vi "Verify.vi"(8 "error in (no error)":errorcluster, 9 "Issuer URI path (component)":string, 10 "Client ID":string, 11 "JSONWebToken in":refnum<class "JSONWebToken.lvclass">) -> (0 "error out":errorcluster, 2 "Valid JWT?":bool, 3 "JSONWebToken out":refnum<class "JSONWebToken.lvclass">)   [LabVIEW 2020, in "JSONWebToken.lvclass"]
doc: "https://openid.net/specs/openid-connect-basic-1_0.html#IDTokenValidation\n\nThe Client MUST validate the ID Token in the Token Response. To do this, the Client can split the ID Token at the period (\".\") characters, take the second segment, and base64url decode it to obtain a JSON object containing the ID Token Claims, which MUST be validated as follows:\n\nThe Issuer Identifier for the OpenID Provider (which is typically obtained during Discovery) MUST exactly match the value of the iss (issuer) Claim.\n\nThe Client MUST validate that the aud (audience) Claim contains its client_id value registered at the Issuer identified by the iss (issuer) Claim as an audience. The ID Token MUST be rejected if the ID Token does not list the Client as a valid audience, or if it contains additional audiences not trusted by the Client.\n\nThe current time MUST be before the time represented by the exp Claim (possibly allowing for some small leeway to account for clock skew).\n\nThe iat Claim can be used to reject tokens that were issued too far away from the current time, limiting the amount of time that nonces need to be stored to prevent attacks. The acceptable range is Client specific.\nIf the acr Claim was requested, the Client SHOULD check that the asserted Claim Value is appropriate. The meaning and processing of acr Claim Values is out of scope for this specification.\n\nWhen a max_age request is made, the Client SHOULD check the auth_time Claim value and request re-authentication if it determines too much time has elapsed since the last End-User authentication."
uses:
  JSONWebToken.lvclass
  JSONWebToken.lvclass/JSONWebToken.ctl
  <vilib>/LabVIEW Open Source Project/OpenSerializer.Base64/Serializer.Base64.lvclass
  LabVIEW-Bits/Cryptographic Services/SHA256/SHA256.lvlib
panel:
  out "date/time claims":T1
  out "Decrypted Text Out":string
  out "signature (encrypted hash)":string
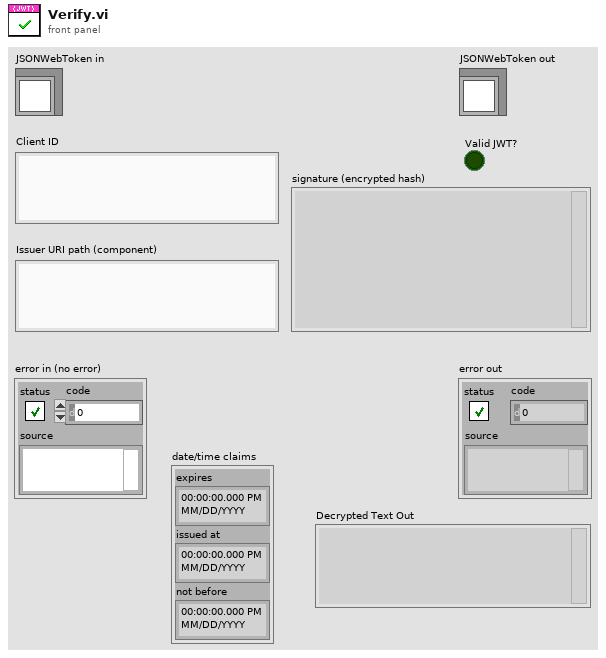
[diagram p1: front panel]
types:
  T1 = cluster{"expires":timestamp, "issued at":timestamp, "not before":timestamp}
  T2 = typedef "header.ctl" = cluster{"alg":string, "jku":string, "jwk":string, "kid":string, "x5u":string, "x5c":string, "x5t":string, "x5t#S256":string, "typ":string, "cty":string, "crit":string, "enc":string}
  T3 = typedef "JSONWebToken.lvclass/JWT registered Claims -- cluster.ctl" = cluster{"iss":string, "sub":string, "aud":string, "exp":i32, "iat":i32, "nbf":i32, "jti":string, "nonce":string, "at_hash":string, "acr":string, "amr":string}
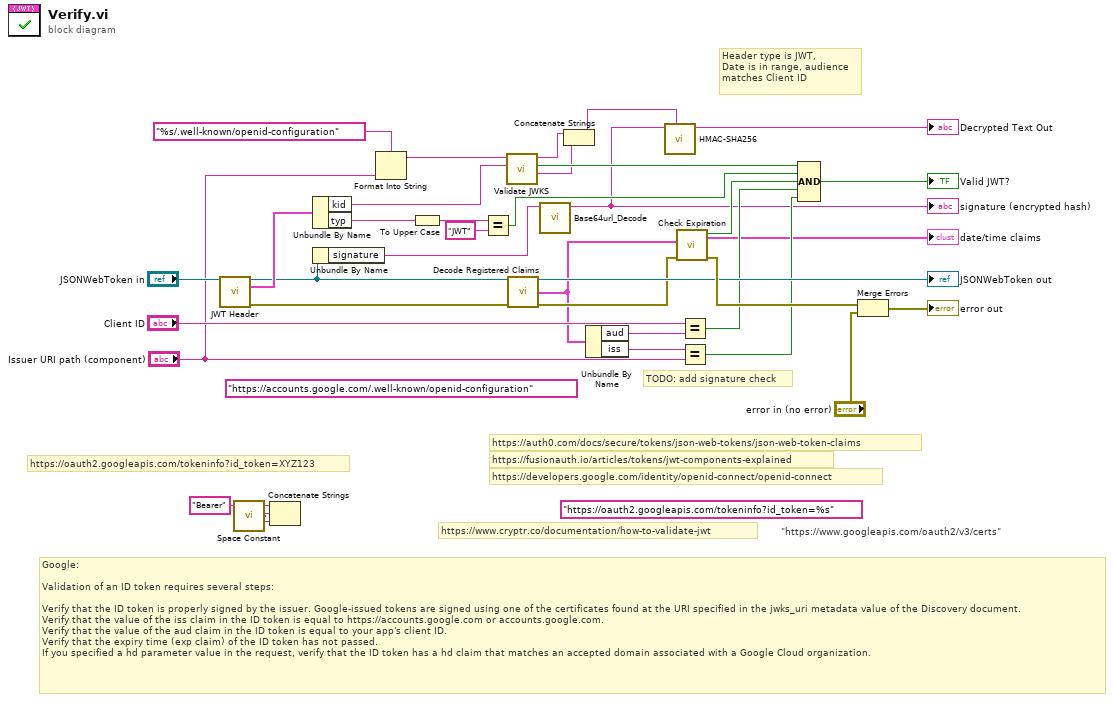
[diagram p0: block diagram]
diagram:
  (unwired) "https://accounts.google.com/.well-known/openid-configuration" ("url")
  (unwired) "https://oauth2.googleapis.com/tokeninfo?id_token=%s"
  # "Header type is JWT,\nDate is in range, audience \nmatches Client ID"
  # "TODO: add signature check"
  # "\"https://www.googleapis.com/oauth2/v3/certs\""
  # "https://oauth2.googleapis.com/tokeninfo?id_token=XYZ123"
  # "https://developers.google.com/identity/openid-connect/openid-connect"
  # "Google:\n\nValidation of an ID token requires several steps:\n\nVerify that the ID token is properly signed by the issuer. Google-issued tokens are signed using one of the certificates found at the URI specified in the jwks_uri metadata value of the Discovery document.\nVerify that the value of the iss claim in the ID token is equal to https://accounts.google.com or accounts.google.com.\nVerify that the value of the aud claim in the ID token is equal to your app's client ID.\nVerify that the expiry time (exp claim) of the ID token has not passed.\nIf you specified a hd parameter value in the request, verify that the ID token has a hd claim that matches an accepted domain associated with a Google Cloud organization."
  # "https://fusionauth.io/articles/tokens/jwt-components-explained"
  # "https://auth0.com/docs/secure/tokens/json-web-tokens/json-web-token-claims"
  # "https://www.cryptr.co/documentation/how-to-validate-jwt"
  n1 = call "JWT Header.vi"("JSONWebToken in"="JSONWebToken in") -> ("JSONWebToken out"=w4:refnum<class "JSONWebToken.lvclass">, "JWT header"=w21:T2, "error out"=w3:errorcluster)  [unwired: 12 in]
  n2 = call <vilib>:"Space Constant.vi"() -> ("String"=w30:string)
  n3 = Concatenate Strings("Bearer" ("path"), w30, w30) -> ()  [unwired: 1 out]
  n4 = Unbundle By Name(w21) -> ("kid"=w19:string, "typ"=w20:string)
  n5 = Unbundle By Name(w4) -> ("signature"=w7:string)
  n6 = Format Into String(format string="%s/.well-known/openid-configuration" ("url"), "Issuer URI path (component)") -> (resulting string=w15:string)  [unwired: 2 in, 1 out]
  n7 = To Upper Case(1:w20) -> (0:w27:string)
  n8 = Equal?(x=w27, y="JWT") -> (x = y?=w24:bool)
  n9 = call "Validate JWKS.vi"("kid"=w19, "jwks_uri"=w15) -> ("e"=w11:string, "kid found?"=w14:bool, "n"=w10:string)  [unwired: 5 in, 2 out]
  n10 = call "Decode Registered Claims.vi"("JSONWebToken in"=w4, "error in (no error)"=w3) -> ("JSONWebToken out"=→"JSONWebToken out":refnum<class "JSONWebToken.lvclass">, "registered claims"=w13:T3, "error out"=w22:errorcluster)  [unwired: 11 in]
  n11 = call <vilib>:"Base64url_Decode.vi"("Base64 URL String"=w7) -> ("Decoded String"=w5:string)  [unwired: 9 in, 1 out]
  "signature (encrypted hash)" <- w5
  n12 = Concatenate Strings(w10, w11) -> (w9:string)
  n13 = Unbundle By Name(w13) -> ("aud"=w26:string, "iss"=w18:string)
  n14 = call "HMAC-SHA256.vi"("Key"=w9, "String to Encode"=w5) -> ("Hash String"=→"Decrypted Text Out":string)  [unwired: 8 in, 1 out]
  n15 = call "Check Expiration.vi"("error in (no error)"=w22, "registered claims"=w13) -> ("error out"=w35:errorcluster, "datetime valid"=w23:bool, "date/time claims"=→"date/time claims":T1)  [unwired: 7 in]
  n16 = Equal?(x="Client ID", y=w26) -> (x = y?=w25:bool)
  n17 = Equal?(x=w18, y="Issuer URI path (component)") -> (x = y?=w17:bool)
  n18 = Compound Arithmetic op=AND(w14, w24, w23, w25, w17) -> (→"Valid JWT?":bool)
  n19 = Merge Errors(w35, "error in (no error)") -> (→"error out":errorcluster)
